vi "Convert Column Index to String.vi"(10 "Column Index (1)":i32=1) -> (2 "Column Letter":string)   [LabVIEW 2017, in "Localization.lvlib" / "Excel Support.lvlib"]
doc: "<B>Description:</B> Converts an Excel Column Index to the appropriuate letter. Index starts at 1.\n1 = A\n26 = Z\n27 = AA\n703 = AAA\n\n<B>Date:</B> 11/2022\n<B>Author:</B> Luke Jarocki, Choose Movement Consulting"
uses:
  Excel Support.lvlib
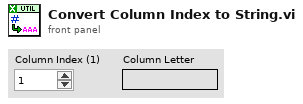
[diagram p1: front panel]
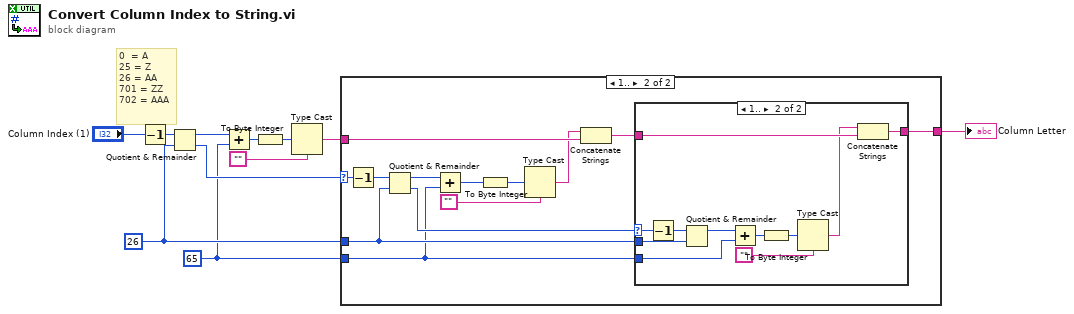
[diagram p0: block diagram]
diagram:
  w2 = 65 ("y")
  w4 = 26 ("y")
  # "0  = A\n25 = Z\n26 = AA\n701 = ZZ\n702 = AAA"
  n1 = Decrement(x="Column Index (1)") -> (x-1=w1:i32)
  n2 = Quotient & Remainder(x=w1, y=w4) -> (x-y*floor(x/y)=w5:i32, floor(x/y)=w7:i32)
  n3 = Add(x=w5, y=w2) -> (x+y=w10:i32)
  n4 = To Byte Integer(number=w10) -> (8bit integer=w8:i8)
  n5 = Type Cast(type="", x=w8) -> (*(type *) &x=w3:string)
  n6 = case shown="1.." w7 {
    selector: w7 -> [_ w23]
    tunnel: w3 -> [w12 w21]
    tunnel: [w12 w18] -> w6
    tunnel: w4 -> [_ w17]
    tunnel: w2 -> [_ w13]
    frame 0, Default {
    }
    frame 1.. {
      n7 = Decrement(x=w23) -> (x-1=w15:i32)
      n8 = Quotient & Remainder(x=w15, y=w17) -> (x-y*floor(x/y)=w16:i32, floor(x/y)=w20:i32)
      n9 = Add(x=w16, y=w13) -> (x+y=w24:i32)
      n10 = To Byte Integer(number=w24) -> (8bit integer=w25:i8)
      n11 = Type Cast(type="", x=w25) -> (*(type *) &x=w14:string)
      n12 = Concatenate Strings(w14, w21) -> (w19:string)
      n13 = case shown="1.." w20 {
        selector: w20 -> [_ w34]
        tunnel: w17 -> [_ w33]
        tunnel: w19 -> [w26 w32]
        tunnel: [w26 w31] -> w18
        tunnel: w13 -> [_ w27]
        frame 0, Default {
        }
        frame 1.. {
          n14 = Decrement(x=w34) -> (x-1=w29:i32)
          n15 = Quotient & Remainder(x=w29, y=w33) -> (x-y*floor(x/y)=w30:i32)  [unwired: 1 out]
          n16 = Add(x=w30, y=w27) -> (x+y=w36:i32)
          n17 = To Byte Integer(number=w36) -> (8bit integer=w35:i8)
          n18 = Type Cast(type="", x=w35) -> (*(type *) &x=w28:string)
          n19 = Concatenate Strings(w28, w32) -> (w31:string)
        }
      }
    }
  }
  "Column Letter" <- w6
